vi "Add WebSockets to palette.vi"() -> ()   [LabVIEW 2013]
uses:
  <vilib>/Palette API/Palette Menu/Public Type Define/Palette type.ctl
  <vilib>/Palette API/Palette Menu/Public Type Define/Item.ctl
  <vilib>/Palette API/Palette Menu/Palette Menu.lvlib
panel:
  out "error out":errorcluster
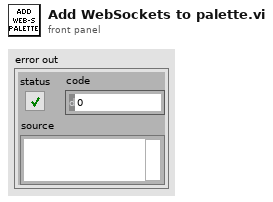
[diagram p1: front panel]
types:
  T1 = typedef "Palette Menu.lvlib/Item.ctl" = cluster{"item path":path, "library path (.lvlib)":path, "use default lvlib palette":bool, "short name":string, "place VI contents":bool, "hide synchronized item":bool, "reserve spot for synch item":bool, "configure when placing VI contents":bool}
  T2 = typedef "Palette Menu.lvlib/Palette type.ctl" = i32
  T3 = typedef "Palette Menu.lvlib/Palette Data.ctl" = cluster{"display name":string, "view format":T4, "palette width":i16, "items":T5, "256 color icon":picture, "B&W color icon":picture, "help information":T6, "palette description":string, "synchronize information":T7}
  T4 = typedef "Palette Menu.lvlib/View Format.ctl" = u16
  T5 = typedef "Palette Menu.lvlib/Items.ctl" = T1[]
  T6 = typedef "Palette Menu.lvlib/Help Info.ctl" = cluster{"help tag":string, "help file path ":path}
  T7 = typedef "Palette Menu.lvlib/Synchronize Info.ctl" = cluster{"synchronize with directory":bool, "synchronize directory path":path}
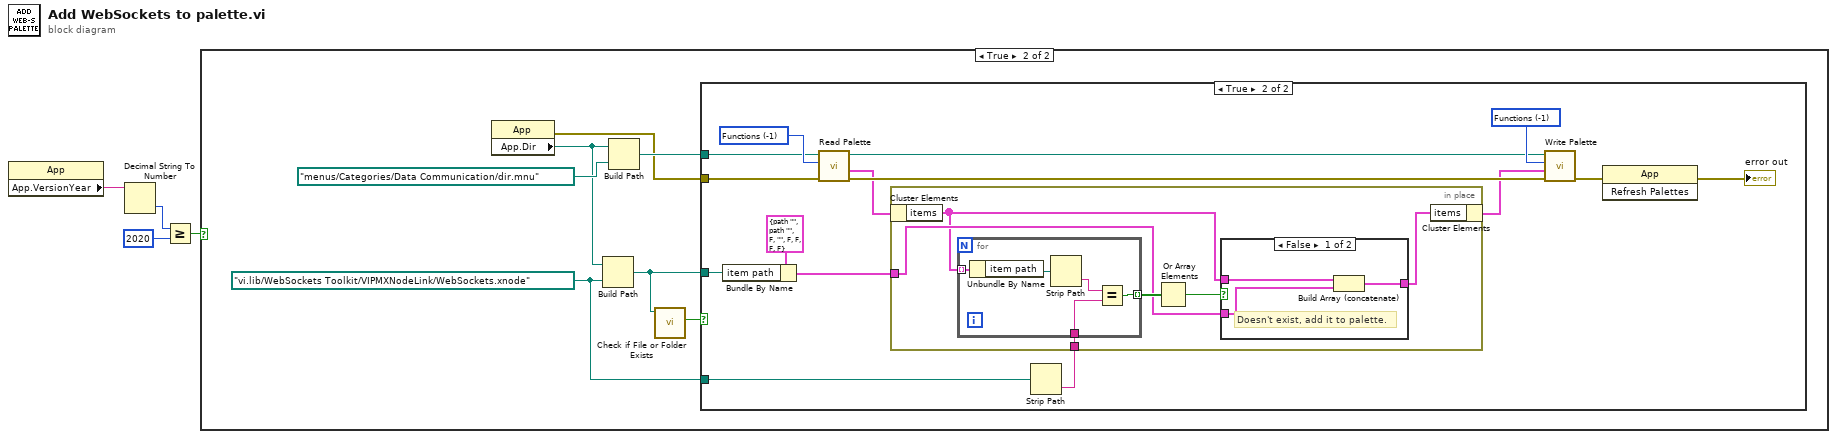
[diagram p0: block diagram]
diagram:
  n1 = property class="App"() -> ("App.VersionYear"=w2:string)  [unwired: 2 in, 2 out]
  n2 = Decimal String To Number(string=w2) -> (number=w4:i32)  [unwired: 2 in, 1 out]
  n3 = Greater Or Equal?(x=w4, y=2020) -> (x >= y?=w1:bool)
  n4 = case shown="True" w1 {
    frame False {
      # "No ops"
    }
    frame True {
      w7 = path "vi.lib/WebSockets Toolkit/VIPMXNodeLink/WebSockets.xnode"
      n5 = property class="App"() -> (error out=w8:errorcluster, "App.Dir"=w9:path)  [unwired: 2 in, 1 out]
      n6 = Build Path(base path=w9, name or relative path=w7) -> (appended path=w6:path)
      n7 = Build Path(base path=w9, name or relative path=path "menus/Categories/Data Communication/dir.mnu") -> (appended path=w10:path)
      n8 = call <vilib>:"Check if File or Folder Exists.vi"("path"=w6) -> ("file or folder exists?"=w5:bool)  [unwired: 8 in, 2 out]
      n9 = case shown="True" w5 {
        tunnel: w10 -> [_ w20]
        tunnel: w8 -> [_ w15]
        tunnel: w7 -> [_ w14]
        tunnel: w6 -> [_ w12]
        frame False {
          # "Xnode doesn't exist, do nothing"
        }
        frame True {
          w21 = T2 -1 items=["Functions"=-1, "Controls"=-2] ("palette type")
          w24 = T2 -1 items=["Functions"=-1, "Controls"=-2] ("palette type")
          n10 = Bundle By Name(cluster=T1 {"item path"=path "", "library path (.lvlib)"=path "", "use default lvlib palette"=FALSE, "short name"="", "place VI contents"=FALSE, "hide synchronized item"=FALSE, "reserve spot for synch item"=FALSE, "configure when placing VI contents"=FALSE} ("Items"), "item path"=w12) -> (w18:T1)
          n11 = call <vilib>:"Read Palette.vi"("error in (no error)"=w15, "palette type"=w21, "palette path"=w20) -> ("error out"=w23:errorcluster, "palette data"=w17:T3, "duplicate palette path"=w22:path)  [unwired: 1 in, 5 out]
          n12 = Strip Path(path=w14) -> (name=w13:string)  [unwired: 1 out]
          n13 = in-place {
            in-place-border: w18 -> [w29]
            in-place-border: w13 -> [w32]
            n14 = in-place-cluster #1(w17) -> ("items"=w27:T5)
            n15 = for {
              tunnel: w27 -> [w41] mode=indexing
              tunnel: w32 -> [w38]
              tunnel: [w37] -> w31 mode=indexing
              n16 = Unbundle By Name(w41) -> ("item path"=w40:path)
              n17 = Strip Path(path=w40) -> (name=w39:string)  [unwired: 1 out]
              n18 = Equal?(x=w39, y=w38) -> (x = y?=w37:bool)
            }
            n19 = Or Array Elements(Boolean array=w31) -> (logical OR=w30:bool)
            n20 = case shown="False" w30 {
              tunnel: w29 -> [w35 _]
              tunnel: [w34 w36] -> w28
              tunnel: w27 -> [w33 w36]
              frame False {
                # "Doesn't exist, add it to palette."
                n21 = Build Array (concatenate)(w33, w35) -> (w34:T5)
              }
              frame True {
                # "Already exists on palette,\ndo nothing."
              }
            }
            n22 = in-place-cluster #1("items"=w28) -> (w16:T3)
          }
          n23 = call <vilib>:"Write Palette.vi"("error in (no error)"=w23, "palette data"=w16, "palette type"=w24, "palette path"=w22) -> ("error out"=w26:errorcluster)  [unwired: 1 in, 6 out]
          n24 = invoke class="App" method="Refresh Palettes"(error in=w26) -> (error out=→"error out":errorcluster)  [unwired: 2 in, 2 out]
        }
      }
    }
  }
